vi "PH_Beamline.Calc Experiment LL State.vi"(0 "i ref in":refnum<vi>, 2 "PA Exit closed":bool, 5 "error in (no error)":errorcluster) -> (14 "i ref out":refnum<vi>, 19 "error out":errorcluster)   [LabVIEW 2014, in "PH_Beamline.lvlib"]
doc: "This VI calculates the experiment laserlab state of the Beamline."
uses:
  PH_Beamline.lvlib
  PH_SystemInformation/PH_SystemInformationEnabling State.ctl
  PH_Common/PH_Common.lvlib
  PH_SystemInformation/PH_SystemInformation.lvlib
  PH_BL-Master/PH_BL-Master.lvlib
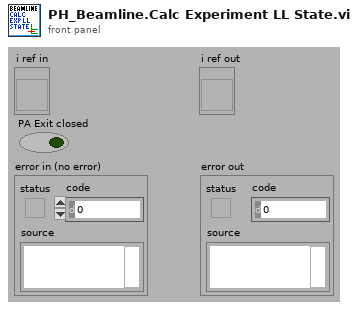
[diagram p1: front panel]
types:
  T1 = typedef "PH_Beamline.lvlib/PH_Beamline.i attribute.ctl" = cluster{"GUI Refs":cluster{"PA ok":refnum<vi>, "MA ok":refnum<vi>, "fs FE ok":refnum<vi>, "ns FE ok":refnum<vi>, "PA ED ok":refnum<vi>, "MAS ok":refnum<vi>, "Booster ok":refnum<vi>, "Mirrortower ok":refnum<vi>, "In.-Box ok":refnum<vi>, "Compressor ok":refnum<vi>, "Experiment LB ok":refnum<vi>, "Experiment LL ok":refnum<vi>, "PHELIX_Beckhoff_Watchdog":refnum<vi>, "Shutters closed":refnum<vi>, "uOPA ok":refnum<vi>, "Vacuum no shotcond Comp LB":refnum<vi>}, "Refs BL MA":refnum<vi>[], "Refs BL MA-IB":refnum<vi>[], "Refs BL fs":refnum<vi>[], "Refs BL PA ED":refnum<vi>[], "Refs BL MAS":refnum<vi>[], "Refs BL Boo":refnum<vi>[], "Refs BL ns":refnum<vi>[], "Refs BL Mirrortower":refnum<vi>[], "Refs BL Compressor":refnum<vi>[], "Refs BL Exp LB":refnum<vi>[], "Radiation Safety":cluster{"Exp Laserbay":cluster{"Ref Op Mode":refnum<vi>, "Ref Laserbay evacuated":refnum<vi>, "Tagname LB evacuated":string, "Shot Mode":T2, "Laserbay evacuated?":i32, "Tagname HV room locked":string, "HV room locked?":i32, "Ref HV room locked":refnum<vi>, "Tagname bridged?":string, "Ref Bridge":refnum<vi>, "I<1E18W/cm²":bool}, "Exp Laserlab":cluster{"Ref Op Mode":refnum<vi>, "Ref Laserlab evacuated":refnum<vi>, "Tagname LL evacuated":string, "Shot Mode":T2, "Laserlab evacuated?":i32, "Tagname bridged?":string, "Ref Bridge":refnum<vi>, "I<1E18W/cm²":bool}}, "Refs BL LL":refnum<vi>[], "PP Igni Heating GUI Refs":refnum<vi>[], "PP Igni Heating Tagnames ":string[], "Refs BL PA":cluster{"undelayed Line before Shutter":refnum<vi>[], "undelayed Line after Shutter":refnum<vi>[], "before Bypass":refnum<vi>[], "delayed Line before Shutter":refnum<vi>[], "delayed Line after Shutter":refnum<vi>[], "before Shutter Input":refnum<vi>[], "after Shutter Input":refnum<vi>[], "Bypass":refnum<vi>[], "before Shutter Exit":refnum<vi>[], "after Shutter Exit":refnum<vi>[], "to MA":refnum<vi>[], "to Lab":refnum<vi>[]}, "BL":cluster{"YLF_BL_Status":i32, "fs_BL_Status":i32, "fs_YLF_BL_Status":i32, "ns_BL_Status":i32, "PA_Input_BL_Status":i32, "PA_UnDelay_BL_Status":i32, "PA_Delay_BL_Status":i32, "PA_BL_Status":i32, "PA_Bypass_BL_Status":i32, "PA_Exit_BL_Status":i32, "PA_LL_BL_Status":i32, "LL_BL_Status":i32, "PA_MA_BL_Status":i32, "MA_Exit_BL_Status":i32, "MA_Z6_BL_Status":i32, "Z6_BL_Status":i32, "MA_LB_BL_Status":i32, "LB_TB2_BL_Status":i32, "PA_before_Bypass_BL_Status":i32, "LB_TB3_BL_Status":i32}, "State Subsystems":cluster{"PA":bool, "MA":bool, "ns FE":bool, "fs FE":bool, "PA ED":bool, "In.-Box":bool, "MAS":bool, "Booster":bool, "Mirrortower":bool, "Compressor":bool, "Experiment LB":bool, "Experiment LL":bool, "uOPA":bool}, "Status Subscriber Information":T3, "Refs BL uOPA":refnum<vi>[], "PA_Input_2_Beam_6PWpGUI not linked?":bool, "PA_Input_Delay_6PGUI not linked?":bool, "Settings":T6}
  T2 = typedef "PH_Beamline.lvlib/PH_Beamline.Operation Mode.ctl" = i32
  T3 = typedef "PH_Beamline.lvlib/PH_Beamline.Status Subscriber Information.ctl" = cluster{"fs Swich YLF":T4, "fs Exit Shutter":T4, "ns Exit Shutter":T4, "PA Input Shutter":T4, "PA PC WP":T4, "PA PC WP 2":T4, "PA Bypass In":T4, "PA Bypass Out":T4, "PA CH 1":T4, "PA delayed":T4, "PA non delayed":T4, "PA Exit Shutter":T4, "PA Switch Lab":T4, "PA Bridge CH Input MA":T4, "MA Diffusor IB":T4, "MA IB Ready":T4, "MA CH 1":T4, "MA CH 2":T4, "MA CH 3":T4, "MA CH 4":T4, "MA Shutter Align Cam":T4, "MA Position MM5":T4, "Calorimeter Switch":T4, "BL Z6 CH 9":T4, "BL Z6 Beamdump":T4, "BL Z6 Shutter":T4, "COS Sensitivity Switch":T4, "Exp LB Shutter":T4, "Exp LB TB 2":T4, "Exp LB TB 3":T4, "PA LL Input CH":T4, "PA LL Output CH":T4, "LL Comp Input Shutter":T4, "LL Comp Output Shutter":T4, "LL Comp FF Shutter":T4, "Exp LL Shutter":T4, "MA IM In IB":T4, "MA IM Out IB":T4, "MA DB In IB":T4, "MA DB Out IB":T4, "Exp LB Shutter Interlock":T4, "Exp LL Shutter Interlock":T4, "MM1 Force Sensor":T4}
  T4 = typedef "PH_BL-Master.lvlib/PH_BL-Master.Status Subscriber Information.ctl" = cluster{"Index of element":i32, "Attributeset":T5}
  T5 = typedef "PH_BL-Master.lvlib/PH_BL-Master.Attribute Set.ctl" = enum16{"Boolean Status Service Subscriber", "Picture Status Service Subscriber"}
  T6 = typedef "PH_Beamline_Chief.lvlib/PH_Beamline_Chief.Settings.ctl" = cluster{"PA Doublepass Mode":bool, "Compressor Vaccuum LB not relevant":bool, "Windowshutter TB2 not relevant":bool, "Windowshutter TB3 not relevant":bool}
  T7 = enum16{"Laser", "PreAmp", "MainAmp", "Exp 1", "Exp 2", "Exp 3", "Exp 4"}[]
  T8 = typedef "PH_SystemInformation.lvlib/PH_SystemInformationEnabling State.ctl" = i32
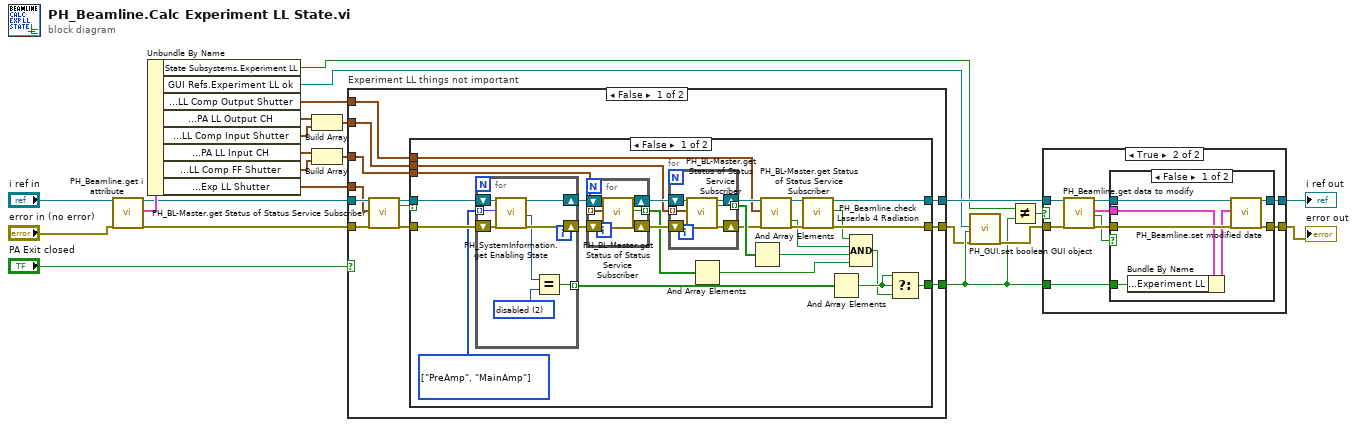
[diagram p0: block diagram]
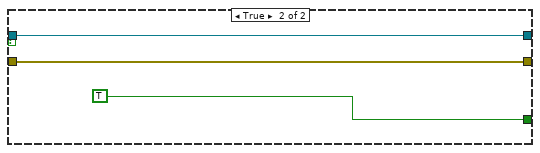
[diagram p4: hidden frame]
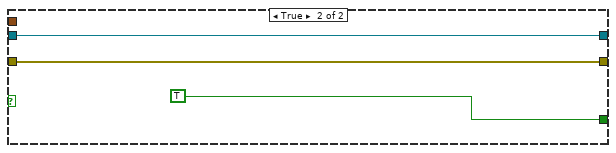
[diagram p5: hidden frame]
diagram:
  n1 = call "PH_Beamline.get i attribute.vi"("i ref in"="i ref in", "error in (no error)"="error in (no error)") -> ("i ref out"=w13:refnum<vi>, "i attribute"=w23:T1, "error out"=w11:errorcluster)  [unwired: 15 in]
  n2 = Unbundle By Name(w23) -> ("State Subsystems.Experiment LL"=w9:bool, "GUI Refs.Experiment LL ok"=w8:refnum<vi>, "Status Subscriber Information.LL Comp Output Shutter"=w1:T4, "Status Subscriber Information.PA LL Output CH"=w4:T4, "Status Subscriber Information.LL Comp Input Shutter"=w3:T4, "Status Subscriber Information.PA LL Input CH"=w7:T4, "Status Subscriber Information.LL Comp FF Shutter"=w6:T4, "Status Subscriber Information.Exp LL Shutter"=w10:T4)
  n3 = Build Array(w4, w3) -> (w2:T4[])
  n4 = Build Array(w7, w6) -> (w5:T4[])
  n5 = case "Experiment LL things not important" shown="False" "PA Exit closed" {
    tunnel: [w35 w87] -> w16
    tunnel: [w34 TRUE] -> w18
    tunnel: [w33 w86] -> w15
    tunnel: w13 -> [w32 w87]
    tunnel: w11 -> [w31 w86]
    tunnel: w10 -> [w27 _]
    tunnel: w5 -> [w26 _]
    tunnel: w2 -> [w25 _]
    tunnel: w1 -> [w24 _]
    frame False {
      n6 = call "PH_BL-Master.get Status of Status Service Subscriber.vi"("i ref in"=w32, "Wanted Status Subscriber Information"=w27, "error in (no error)"=w31) -> ("i ref out"=w30:refnum<vi>, "off/false/out?"=w28:bool, "error out"=w29:errorcluster)  [unwired: 11 in, 3 out]
      n7 = case "Experiment LL things not important" shown="False" w28 {
        tunnel: w30 -> [w56 w84]
        tunnel: [w61 w84] -> w35
        tunnel: w29 -> [w55 w83]
        tunnel: [w60 w83] -> w33
        tunnel: [w53 TRUE] -> w34
        tunnel: w26 -> [w38 _]
        tunnel: w25 -> [w37 _]
        tunnel: w24 -> [w36 _]
        frame False {
          w54 = T7 [enum."PreAmp", enum."MainAmp"] items=["Laser", "PreAmp", "MainAmp", "Exp 1", "Exp 2", "Exp 3", "Exp 4"]
          n8 = for {
            shift-right: [w80] -> w45
            shift-left: w56 -> [w81]
            shift-right: [w78] -> w43
            shift-left: w55 -> [w79]
            tunnel: w54 -> [w77] mode=indexing
            tunnel: [w74] -> w58 mode=indexing
            w75 = T8 2 items=["no info", "not disabled", "disabled"] ("y")
            n9 = call "PH_SystemInformation.get Enabling State.vi"("i ref in"=w81, "Wanted State"=w77, "error in (no error)"=w79) -> ("i ref out"=w80:refnum<vi>, "Enabling State"=w76:T8, "error out"=w78:errorcluster)  [unwired: 14 in]
            n10 = Equal?(x=w76, y=w75) -> (x = y?=w74:bool)
          }
          n11 = for {
            tunnel: [w63] -> w41 mode=indexing
            tunnel: w38 -> [w62] mode=indexing
            shift-right: [w66] -> w44
            shift-left: w45 -> [w67]
            shift-right: [w64] -> w42
            shift-left: w43 -> [w65]
            n12 = call "PH_BL-Master.get Status of Status Service Subscriber.vi"("i ref in"=w67, "Wanted Status Subscriber Information"=w62, "error in (no error)"=w65) -> ("i ref out"=w66:refnum<vi>, "on/true/in?"=w63:bool, "error out"=w64:errorcluster)  [unwired: 11 in, 3 out]
          }
          n13 = for {
            tunnel: [w68] -> w59 mode=indexing
            tunnel: w37 -> [w69] mode=indexing
            shift-right: [w72] -> w49
            shift-left: w44 -> [w71]
            shift-right: [w73] -> w51
            shift-left: w42 -> [w70]
            n14 = call "PH_BL-Master.get Status of Status Service Subscriber.vi"("i ref in"=w71, "Wanted Status Subscriber Information"=w69, "error in (no error)"=w70) -> ("i ref out"=w72:refnum<vi>, "off/false/out?"=w68:bool, "error out"=w73:errorcluster)  [unwired: 11 in, 3 out]
          }
          n15 = And Array Elements(Boolean array=w41) -> (logical AND=w40:bool)
          n16 = And Array Elements(Boolean array=w59) -> (logical AND=w52:bool)
          n17 = call "PH_BL-Master.get Status of Status Service Subscriber.vi"("i ref in"=w49, "Wanted Status Subscriber Information"=w36, "error in (no error)"=w51) -> ("i ref out"=w48:refnum<vi>, "off/false/out or on/true/in?"=w46:bool, "error out"=w50:errorcluster)  [unwired: 11 in, 3 out]
          n18 = call "PH_Beamline.check Laserlab 4 Radiation.vi"("i ref in"=w48, "error in"=w50) -> ("i ref out"=w61:refnum<vi>, "Laserlab save concerning Radiation"=w47:bool, "error out"=w60:errorcluster)  [unwired: 15 in]
          n19 = And Array Elements(Boolean array=w58) -> (logical AND=w57:bool)
          n20 = Compound Arithmetic op=AND(w47, w46, w52, w40) -> (w39:bool)
          n21 = Select(t=w57, s=w57, f=w39) -> (s? t:f=w53:bool)
        }
        frame True {
        }
      }
    }
    frame True {
    }
  }
  n22 = call "PH_GUI.set boolean GUI object.vi"("Boolean Knob GUI Ref"=w8, "Value"=w18, "error in (no error)"=w15) -> ("error out"=w20:errorcluster)  [unwired: 16 in]
  n23 = Not Equal?(x=w9, y=w18) -> (x != y?=w22:bool)
  n24 = case shown="True" w22 {
    tunnel: [w89 w94] -> w21
    tunnel: [w88 w93] -> w19
    tunnel: w18 -> [_ w92]
    tunnel: w20 -> [w88 w91]
    tunnel: w16 -> [w89 w90]
    frame False {
    }
    frame True {
      n25 = call "PH_Beamline.get data to modify.vi"("i ref in"=w90, "error in (no error)"=w91) -> ("i ref out"=w97:refnum<vi>, "i attribute"=w95:T1, "timed out"=w96:bool, "error out"=w98:errorcluster)  [unwired: 14 in]
      n26 = case shown="False" w96 {
        tunnel: w98 -> [w105 w106]
        tunnel: w97 -> [w104 w107]
        tunnel: [w103 w106] -> w93
        tunnel: [w102 w107] -> w94
        tunnel: w95 -> [w101 _]
        tunnel: w92 -> [w99 _]
        frame False {
          n27 = Bundle By Name(cluster=w101, "State Subsystems.Experiment LL"=w99) -> (w100:T1)
          n28 = call "PH_Beamline.set modified data.vi"("i ref in"=w104, "i attribute"=w100, "error in (no error)"=w105) -> ("i ref out"=w102:refnum<vi>, "error out"=w103:errorcluster)  [unwired: 15 in]
        }
        frame True {
        }
      }
    }
  }
  "i ref out" <- w21
  "error out" <- w19
